vi "Data_logging.vi"() -> ()   [LabVIEW 2016]
uses:
  adsorbed_cluster.ctl
  File_name.ctl
  EOS.ctl
  auxiliary_cluster.ctl
panel:
  in  "Auxiliary Data":T1 {"EOS" items=["Ideal", "CH4_van_der_Waal", "CH4_Redlich_Kwong", "CO2_van_der_Waal", "CO2_Redlich_Kwong", ""]}
  in  "File Name":T3
  in  "Adsorbed":T4 {"Pressure (barg)" scale=0.0..70.0}
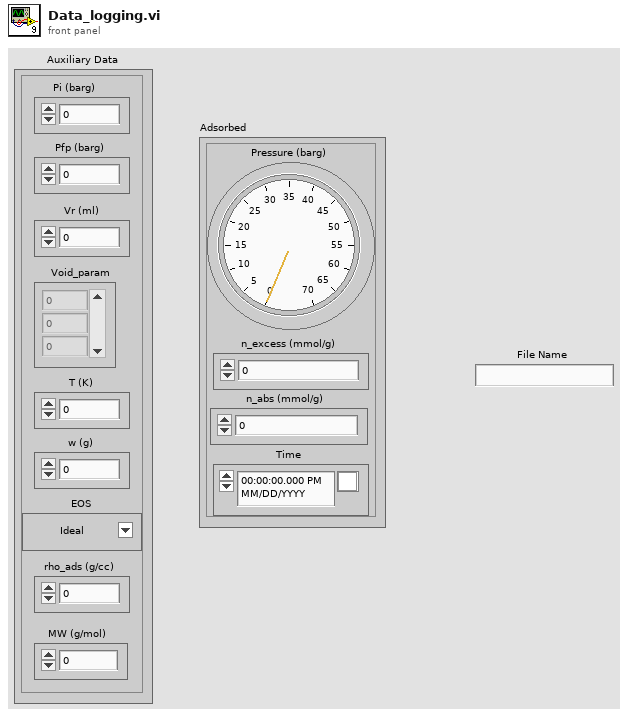
[diagram p1: front panel]
types:
  T1 = typedef "auxiliary_cluster.ctl" = cluster{"Pi (barg)":dbl, "Pfp (barg)":dbl, "Vr (ml)":dbl, "T (K)":dbl, "w (g)":dbl, "Void_param":dbl[], "EOS":T2, "rho_ads (g/cc)":dbl, "MW (g/mol)":dbl}
  T2 = typedef "EOS.ctl" = u16
  T3 = typedef "File_name.ctl" = string
  T4 = typedef "adsorbed_cluster.ctl" = cluster{"Time":timestamp, "Pressure (barg)":dbl, "n_excess (mmol/g)":dbl, "n_abs (mmol/g)":dbl}
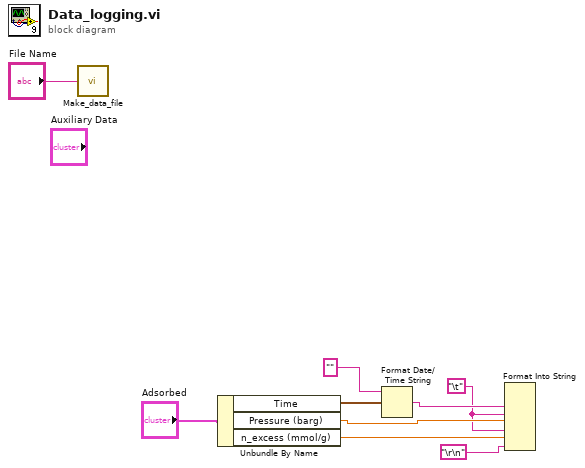
[diagram p0: block diagram]
diagram:
  w4 = "\t"
  n1 = call "Make_data_file.vi"("File Name"="File Name") -> ()  [unwired: 1 out]
  n2 = Unbundle By Name("Adsorbed") -> ("Time"=w7:timestamp, "Pressure (barg)"=w5:dbl, "n_excess (mmol/g)"=w3:dbl)
  n3 = Format Date/Time String(time format string (%c)="", seconds (now)=w7) -> (date/time string=w6:string)  [unwired: 1 in]
  n4 = Format Into String(w6, w4, w5, w4, w3, "\r\n") -> ()  [unwired: 3 in, 2 out]
